vi "subHamamatsu_Initialization.vi"(6 "Camera Ctrl":T2={"Chosen Camera"=0, "ROI selection"=0, "Live"=FALSE, "ROI define"=FALSE, "Snap"=FALSE, "ROI update"=FALSE, "ROI previous "=FALSE, "ROI"={"Bin"=2, "ROI"={"x offset"=256, "y offset"=256, "x width"=512, "y width"=512}}, "Exposure (ms)"=100.0, "Symmetrical"=FALSE, "Autoscale"=TRUE, "Scale"={"Scale.Min"=0, "Scale.Max"=6038}} {"Scale"."Scale.Max" min=1 max=5000 step=1; "Scale"."Scale.Min" min=1 max=5000 step=1; "Exposure (ms)" min=1.0 max=5000.0 step=1.0; "ROI"."ROI"."x offset" min=1 max=512 step=1; "ROI"."ROI"."y offset" min=1 max=512 step=1; "ROI"."ROI"."x width" min=1 max=512 step=1; "ROI"."ROI"."y width" min=1 max=512 step=1; "ROI"."Bin" items=["1x1"=1, "2x2"=2, "4x4"=4]; "ROI selection" items=["Full ROI", "Central quad", "Confocal"]; "Chosen Camera" items=["Left", "Right"]}, 8 "error in (no error)":errorcluster {"code" format="%.0x"}, 11 "Camera Setting":T1={"Camera Output triger mode setiting"={"Mode"=3, "Polarity"=2, "Period"=0.0005, "Delay"=0.0}, "Camera timing port for trigering"=enum."3"} {"Camera Output triger mode setiting"."Polarity" items=["Negative"=1, "Positive"=2]; "Camera Output triger mode setiting"."Mode" items=["Low"=1, "Global Exposure"=2, "Programmable"=3, "Trigger Ready"=4, "High"=5]}) -> (0 "error out":errorcluster, 1 "Chosen Camera":u32(ring) items=["Left", "Right"], 3 "Handle out":u32, 4 "Camera Info":T3={"Camera Details Array"=[{"Model"="C11440-22C", "Camera ID"="S/N: 003223", "Firmware"="3.20.A"}], "Handle"=0, "Camera in use "={"Model"="C11440-22C", "Camera ID"="S/N: 003223", "Bits"=16}}, 5 "Number Of Cameras":u32=2, 7 "Camera initialized":bool[](array[boolean]))   [LabVIEW 2015]
panel:
  # "Left Camera"
  # "Right Camera"
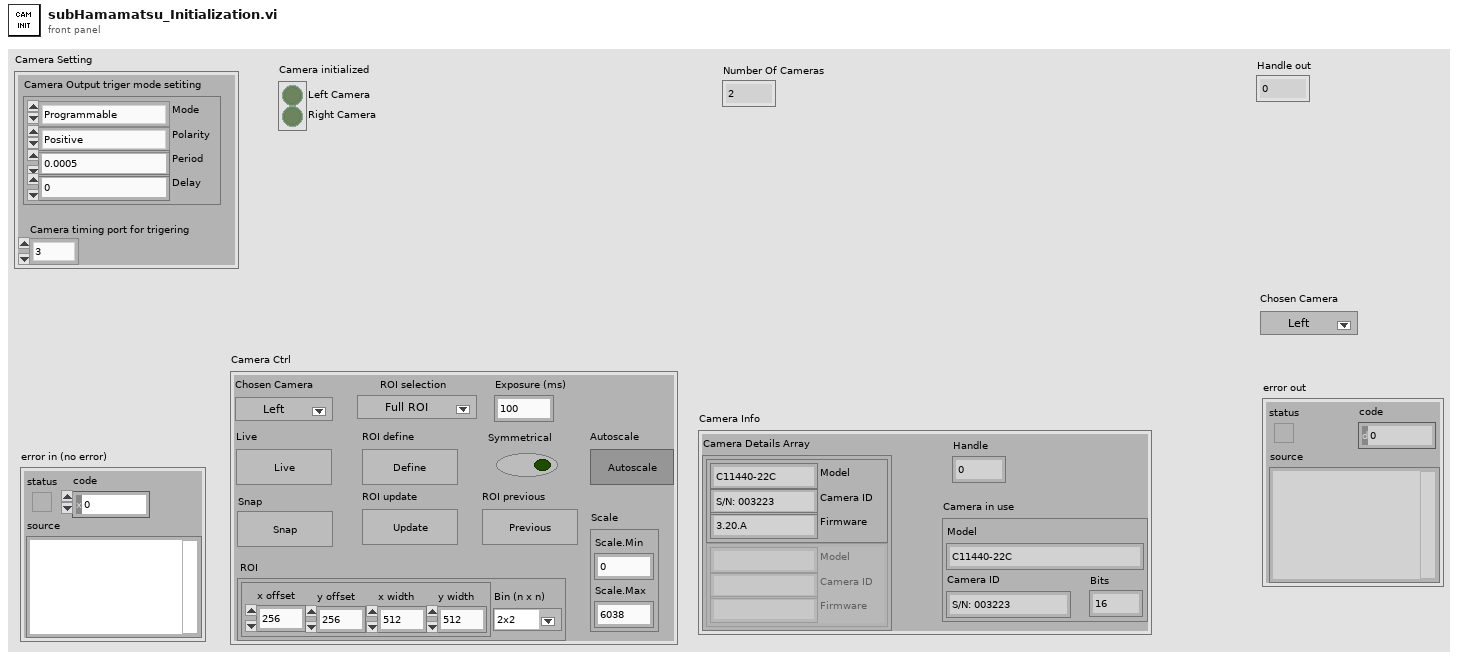
[diagram p1: front panel]
types:
  T1 = cluster{"Camera Output triger mode setiting":cluster{"Mode":u32, "Polarity":u32, "Period":dbl, "Delay":dbl}, "Camera timing port for trigering":enum16{"1", "2", "3"}}
  T2 = cluster{"Chosen Camera":u32, "ROI selection":u16, "Live":bool, "ROI define":bool, "Snap":bool, "ROI update":bool, "ROI previous ":bool, "ROI":cluster{"Bin":u16, "ROI":cluster{"x offset":i32, "y offset":i32, "x width":i32, "y width":i32}}, "Exposure (ms)":dbl, "Symmetrical":bool, "Autoscale":bool, "Scale":cluster{"Scale.Min":i32, "Scale.Max":i32}}
  T3 = cluster{"Camera Details Array":cluster{"Model":string, "Camera ID":string, "Firmware":string}[], "Handle":u32, "Camera in use ":cluster{"Model":string, "Camera ID":string, "Bits":i32}}
  T4 = cluster{"Model":string, "Camera ID":string, "Firmware":string}[]
  T5 = cluster{"Model":string, "Camera ID":string, "Bits":i32}
  T6 = cluster{"Bin":u16, "ROI":cluster{"x offset":i32, "y offset":i32, "x width":i32, "y width":i32}}
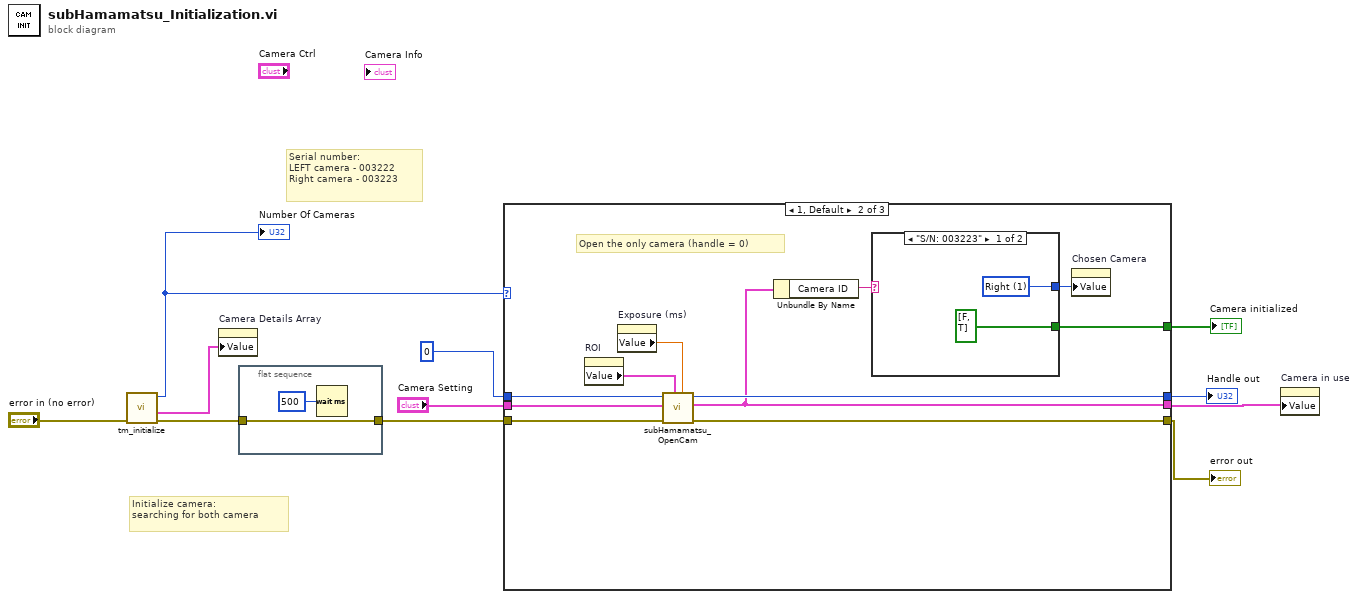
[diagram p0: block diagram]
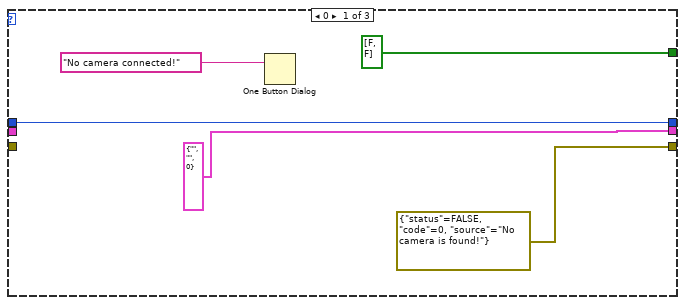
[diagram p2: hidden frame]
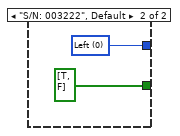
[diagram p3: hidden frame]
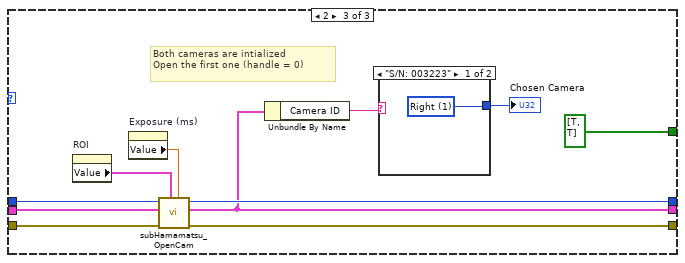
[diagram p4: hidden frame]
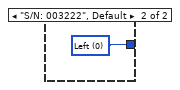
[diagram p5: hidden frame]
diagram:
  # "Initialize camera:\nsearching for both camera"
  # "Serial number:\nLEFT camera - 003222\nRight camera - 003223"
  n1 = call <userlib>:"tm_initialize.vi"("error in (no error)"="error in (no error)") -> ("error out"=w10:errorcluster, "Camera Details Array"=w5:T4, "Number Of Cameras"=w7:u32)  [unwired: 7 in, 1 out]
  "Number Of Cameras" <- w7
  n2 = property on="Camera Details Array" class="Arr (strict)"("Value"=w5) -> ()  [unwired: 2 in, 2 out]
  n3 = flat-sequence {
    tunnel: w10 -> [w12]
    tunnel: [w12] -> w11
    frame #0 {
      n4 = Wait (ms)(milliseconds to wait=u32 500) -> ()  [unwired: 1 out]
    }
  }
  n5 = case shown="1, Default" w7 {
    tunnel: w11 -> [_ w28 w44]
    tunnel: [errorcluster {"status"=FALSE, "code"=0, "source"="No camera is found!"} ("camera \ninitialization\nerror") w27 w43] -> w9
    tunnel: [bool[] [FALSE, FALSE] w29 bool[] [TRUE, TRUE]] -> w6
    tunnel: "Camera Setting" -> [_ w25 w42]
    tunnel: u32 0 ("Handle in") -> [w16 w26 w41]
    tunnel: [w16 w22 w40] -> w2
    tunnel: [T5 {"Model"="", "Camera ID"="", "Bits"=0} ("Camera in use") w20 w37] -> w1
    frame 0 {
      n6 = One Button Dialog(message="No camera connected!") -> ()  [unwired: 1 in, 1 out]
    }
    frame 1, Default {
      # "Open the only camera (handle = 0)"
      n7 = property on="ROI" class="Clust (strict)"() -> ("Value"=w24:T6)  [unwired: 2 in, 2 out]
      n8 = property on="Exposure (ms)" class="DigNum (strict)"() -> ("Value"=w23:dbl)  [unwired: 2 in, 2 out]
      n9 = call "subHamamatsu_OpenCam.vi"("Exposure (ms)"=w23, "ROI"=w24, "error in (no error)"=w28, "Camera Setting"=w25, "Handle in"=w26) -> ("error out"=w27:errorcluster, "Camera in use"=w20:T5, "Handle out"=w22:u32)  [unwired: 4 in]
      n10 = Unbundle By Name(w20) -> ("Camera ID"=w21:string)
      n11 = case shown="\"S/N: 003223\"" w21 {
        tunnel: [bool[] [FALSE, TRUE] bool[] [TRUE, FALSE]] -> w29
        tunnel: [w30 w32] -> w19
        frame "S/N: 003223" {
          w30 = u32 1 items=["Left", "Right"] ("Chosen Camera")
        }
        frame "S/N: 003222", Default {
          w32 = u32 0 items=["Left", "Right"] ("Chosen Camera")
        }
      }
      n12 = property on="Chosen Camera" class="Ring (strict)"("Value"=w19) -> ()  [unwired: 2 in, 2 out]
    }
    frame 2 {
      # "Both cameras are intialized\nOpen the first one (handle = 0)"
      n13 = property on="ROI" class="Clust (strict)"() -> ("Value"=w39:T6)  [unwired: 2 in, 2 out]
      n14 = property on="Exposure (ms)" class="DigNum (strict)"() -> ("Value"=w38:dbl)  [unwired: 2 in, 2 out]
      n15 = call "subHamamatsu_OpenCam.vi"("Exposure (ms)"=w38, "ROI"=w39, "error in (no error)"=w44, "Camera Setting"=w42, "Handle in"=w41) -> ("error out"=w43:errorcluster, "Camera in use"=w37:T5, "Handle out"=w40:u32)  [unwired: 4 in]
      n16 = Unbundle By Name(w37) -> ("Camera ID"=w36:string)
      n17 = case shown="\"S/N: 003223\"" w36 {
        tunnel: [w45 w46] -> w34
        frame "S/N: 003223" {
          w45 = u16 1 items=["Left", "Right"] ("Choose Camera")
        }
        frame "S/N: 003222", Default {
          w46 = u16 0 items=["Left", "Right"] ("Choose Camera")
        }
      }
      "Chosen Camera" <- w34
    }
  }
  "error out" <- w9
  "Camera initialized" <- w6
  "Handle out" <- w2
  n18 = property on="Camera in use" class="Clust (strict)"("Value"=w1) -> ()  [unwired: 2 in, 2 out]
